vi "(SubVI) Convert CB idx to talents.vi"(2 "index":i32, 3 "Talent order CB":string[](array[string])) -> (0 "Talent 2":string, 1 "Talent 1":string)   [LabVIEW 2024]
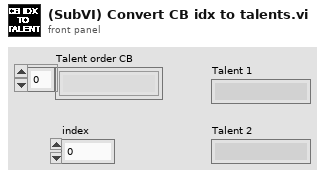
[diagram p1: front panel]
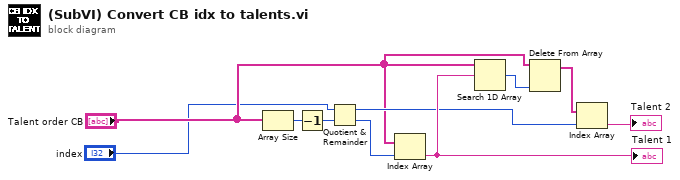
[diagram p0: block diagram]
diagram:
  n1 = Array Size(array="Talent order CB") -> (size(s)=w1:i32)
  n2 = Decrement(x=w1) -> (x-1=w2:i32)
  n3 = Quotient & Remainder(x="index", y=w2) -> (x-y*floor(x/y)=w7:i32, floor(x/y)=w6:i32)
  n4 = Index Array(array="Talent order CB", index=w6) -> (element=w10:string)
  "Talent 1" <- w10
  n5 = Search 1D Array(1D array="Talent order CB", element=w10) -> (index of element=w4:i32)  [unwired: 1 in]
  n6 = Delete From Array(array="Talent order CB", index=w4) -> (array with subset deleted=w8:string[])  [unwired: 1 in, 1 out]
  n7 = Index Array(array=w8, index=w7) -> (element=→"Talent 2":string)
